vi "dfd_Numeric is Even.vi"(1 "N":i32=2) -> (0 "even ?":bool)   [LabVIEW 2017, in "NI_DigFilterLicensed.lvlib"]
doc: "Checks whether the numerator order is even or not."
uses:
  <vilib>/addons/Digital Filter Design/NI_DigFilterLicensed.lvlib
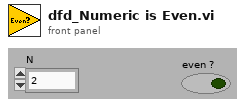
[diagram p1: front panel]
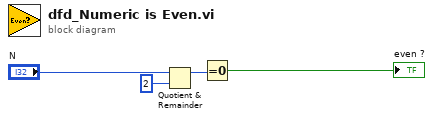
[diagram p0: block diagram]
diagram:
  n1 = Quotient & Remainder(x="N", y=2) -> (x-y*floor(x/y)=w3:i32)  [unwired: 1 out]
  n2 = Equal To 0?(x=w3) -> (x = 0?=→"even ?":bool)
